vi "Untitled 4.vi"() -> ()   [LabVIEW 2017]
panel:
  out "y 2":u16 format="%x"
  in  "y":u16
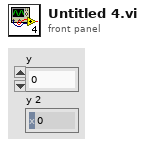
[diagram p1: front panel]
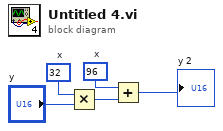
[diagram p0: block diagram]
diagram:
  w3 = u16 96  # x
  w5 = u16 32  # x
  n1 = Multiply(x=w5, y="y") -> (x*y=w4:u16)
  n2 = Add(x=w3, y=w4) -> (x+y=→"y 2":u16)
